vi "WriteDO.vi"(8 "error in (no error)":errorcluster, 9 "DOValue":bool, 10 "DOBit":u8, 11 "DIO in":refnum<class "DIO.lvclass">) -> (0 "error out":errorcluster, 3 "DIO out":refnum<class "DIO.lvclass">)   [LabVIEW 2024, in "DIO Actor.lvlib" / "DIO.lvclass"]
uses:
  DIO.lvclass
  DIO.lvclass/DIO.ctl
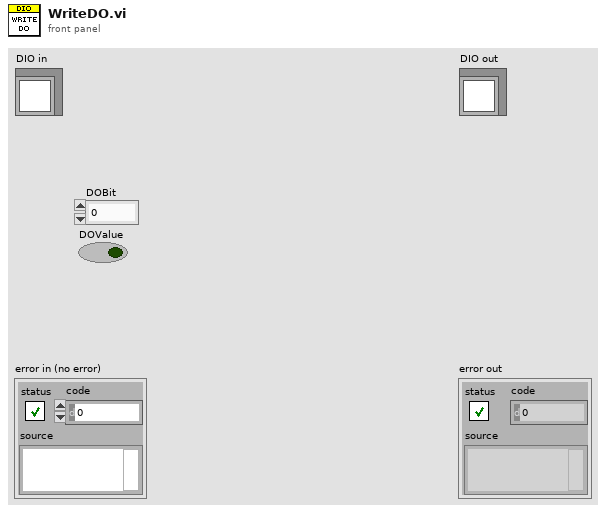
[diagram p1: front panel]
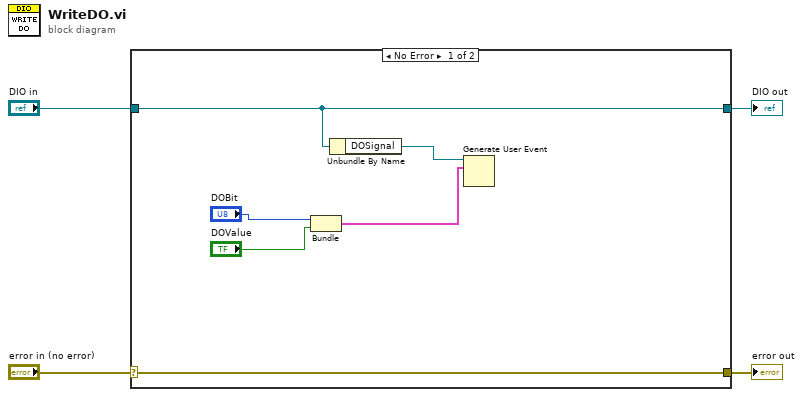
[diagram p0: block diagram]
diagram:
  n1 = case shown="No Error" "error in (no error)" {
    selector: "error in (no error)" -> [w10 w12]
    tunnel: [w10 w12] -> w3
    tunnel: [w9 w11] -> w1
    tunnel: "DIO in" -> [w9 w11]
    frame No Error {
      n2 = Bundle("DOBit"="DOBit", "DOValue"="DOValue") -> (w5:cluster{"DOBit":u8, "DOValue":bool})  [unwired: 1 in]
      n3 = Unbundle By Name(w9) -> ("DOSignal"=w8:refnum<user-event>)
      n4 = Generate User Event(user event=w8, event data cluster=w5) -> ()  [unwired: 2 in, 2 out]
    }
    frame Error {
    }
  }
  "error out" <- w3
  "DIO out" <- w1
